vi "ComposeCustomBlendMode.vi"(4 "DstAlphaFactor":T3=enum."SDL_BLENDFACTOR_ZERO", 5 "DstColorFactor":T3=enum."SDL_BLENDFACTOR_ZERO", 6 "SrcAlphaFactor":T3=enum."SDL_BLENDFACTOR_ZERO", 7 "SrcColorFactor":T3=enum."SDL_BLENDFACTOR_ZERO", 8 "No Error":errorcluster, 10 "AlphaOperation":T2=enum."SDL_BLENDOPERATION_ADD", 11 "ColorOperation":T2=enum."SDL_BLENDOPERATION_ADD") -> (0 "error out":errorcluster, 3 "BlendMode":T1 items=["SDL_BLENDMODE_NONE"=0, "SDL_BLENDMODE_BLEND"=1, "SDL_BLENDMODE_BLEND_PREMULTIPLIED"=16, "SDL_BLENDMODE_ADD"=2, "SDL_BLENDMODE_ADD_PREMULTIPLIED"=32, "SDL_BLENDMODE_MOD"=4, "SDL_BLENDMODE_MUL"=8, "SDL_BLENDMODE_INVALID"=2147483647])   [LabVIEW 2024, in "SDL3.lvlib" / "Blendmode.lvlib"]
doc: "<B>Summary</B>\nCompose a custom blend mode for renderers.\n\n<B>Remarks</B>\nThe functions SDL_SetRenderDrawBlendMode and SDL_SetTextureBlendMode accept the SDL_BlendMode returned by this function if the renderer supports it.\n\nA blend mode controls how the pixels from a drawing operation (source) get combined with the pixels from the render target (destination). First, the components of the source and destination pixels get multiplied with their blend factors. Then, the blend operation takes the two products and calculates the result that will get stored in the render target.\n\nExpressed in pseudocode, it would look like this:\n\ndstRGB = colorOperation(srcRGB * srcColorFactor, dstRGB * dstColorFactor);\ndstA = alphaOperation(srcA * srcAlphaFactor, dstA * dstAlphaFactor);\nWhere the functions colorOperation(src, dst) and alphaOperation(src, dst) can return one of the following:\n\nsrc + dst\nsrc - dst\ndst - src\nmin(src, dst)\nmax(src, dst)\nThe red, green, and blue components are always multiplied with the first, second, and third components of the SDL_BlendFactor, respectively. The fourth component is not used.\n\nThe alpha component is always multiplied with the fourth component of the SDL_BlendFactor. The other components are not used in the alpha calculation.\n\nSupport for these blend modes varies for each renderer. To check if a specific SDL_BlendMode is supported, create a renderer and pass it to either SDL_SetRenderDrawBlendMode or SDL_SetTextureBlendMode. They will return with an error if the blend mode is not supported.\n\nThis list describes the support of custom blend modes for each renderer. All renderers support the four blend modes listed in the SDL_BlendMode enumeration.\n\ndirect3d: Supports all operations with all factors. However, some factors produce unexpected results with SDL_BLENDOPERATION_MINIMUM and SDL_BLENDOPERATION_MAXIMUM.\ndirect3d11: Same as Direct3D 9.\nopengl: Supports the SDL_BLENDOPERATION_ADD operation with all factors. OpenGL versions 1.1, 1.2, and 1.3 do not work correctly here.\nopengles2: Supports the SDL_BLENDOPERATION_ADD, SDL_BLENDOPERATION_SUBTRACT, SDL_BLENDOPERATION_REV_SUBTRACT operations with all factors.\npsp: No custom blend mode support.\nsoftware: No custom blend mode support.\nSome renderers do not provide an alpha component for the default render target. The SDL_BLENDFACTOR_DST_ALPHA and SDL_BLENDFACTOR_ONE_MINUS_DST_ALPHA factors do not have an effect in this case."
uses:
  Blendmode.lvlib
  BlendFactor--enum.ctl
  BlendOperation--enum.ctl
  BlendMode--ring.ctl
  Lib/SDL3-32.dll
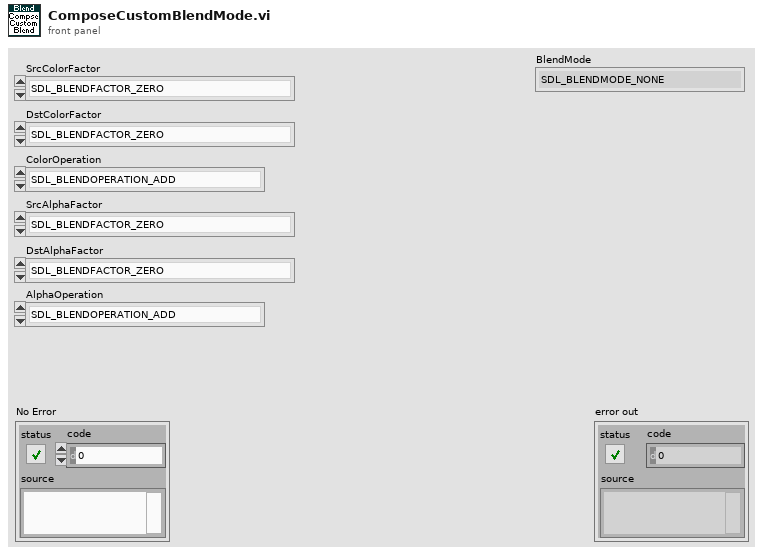
[diagram p1: front panel]
types:
  T1 = typedef "SDL3.lvlib/Blendmode.lvlib/BlendMode--ring.ctl" = u32
  T2 = typedef "SDL3.lvlib/Blendmode.lvlib/BlendOperation--enum.ctl" = enum32{"LV_INVALID", "SDL_BLENDOPERATION_ADD", "SDL_BLENDOPERATION_SUBTRACT", "SDL_BLENDOPERATION_REV_SUBTRACT", "SDL_BLENDOPERATION_MINIMUM", "SDL_BLENDOPERATION_MAXIMUM"}
  T3 = typedef "SDL3.lvlib/Blendmode.lvlib/BlendFactor--enum.ctl" = enum32{"LV_INVALID", "SDL_BLENDFACTOR_ZERO", "SDL_BLENDFACTOR_ONE", "SDL_BLENDFACTOR_SRC_COLOR", "SDL_BLENDFACTOR_ONE_MINUS_SRC_COLOR", "SDL_BLENDFACTOR_SRC_ALPHA", "SDL_BLENDFACTOR_ONE_MINUS_SRC_ALPHA", " SDL_BLENDFACTOR_DST_COLOR", "SDL_BLENDFACTOR_ONE_MINUS_DST_COLOR", "SDL_BLENDFACTOR_DST_ALPHA", "SDL_BLENDFACTOR_ONE_MINUS_DST_ALPHA"}
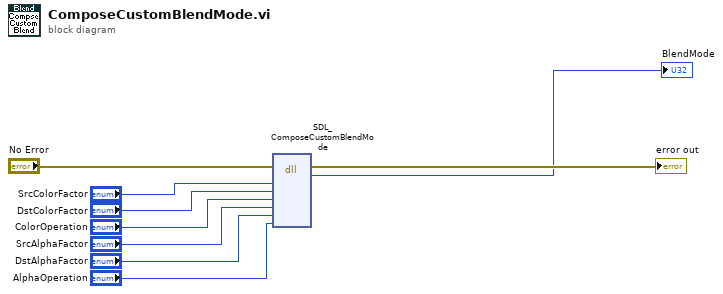
[diagram p0: block diagram]
diagram:
  n1 = dll-call lib="C:/Users/Thomas/Documents/Projects/LV-SDL3/Lib/SDL3-*.*" fn="SDL_ComposeCustomBlendMode"(error in="No Error", "srcColorFactor"="SrcColorFactor", "dstColorFactor"="DstColorFactor", "colorOperation"="ColorOperation", "srcAlphaFactor"="SrcAlphaFactor", "dstAlphaFactor"="DstAlphaFactor", "alphaOperation"="AlphaOperation") -> (error out=→"error out":errorcluster, "return type"=→"BlendMode":u32)  [unwired: 8 in, 1 out]
